vi "CFTS-Globals.vi"() -> ()   [LabVIEW 2020]
panel:
  in  "Version":string="3.5"
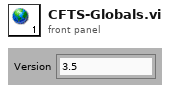
[diagram p1: front panel]
diagram:
